vi "Benchmarking Asynchronous Calls.vi"() -> ()   [LabVIEW 2016]
doc: "This example requests web pages from the specified servers using an HTTP Get request and records how long the requests take. This example demonstrates and compares four different design patterns that accomplish this task:\n\n* Call By Reference node inside a For Loop to sequentially call the target VI\n* Call By Reference node inside a Parallel For Loop to allow some calls to execute in parallel depending on the number of CPU cores\n* Run VI method to execute all calls in parallel\n* Asynchronously calling VIs using the Start Asynchronous Call node to execute all calls in parallel\n\nIn general, if an application is I/O bound (ex: communication over the network), the parallel call approaches perform better. The default behavior of the Parallel For loop will run frames in parallel based on the number of CPU cores. The Run VI method and asynchronous call patterns allow a user to define the amount of parallelism at run time. \n\nIf an application is local CPU bound, the Parallel For Loop approach will perform the best. It utilizes the number of CPU cores and has less overhead when compared to the Run VI method and the asynchronous call pattern.\n\nThe actual performance results for this example depend largely on the computer and network connection.\n\nThe asynchronous call pattern and the Run VI method require overhead to allow the run-time defined parallelism. This overhead is negligible when compared to the I/O usage as in this example. The asynchronous call pattern has less overhead than the Run VI method. Depending on the application, the asynchronous call pattern might require LabVIEW to open fewer VI references and is more efficient when passing parameters to and from the target VI. The asynchronous call pattern also has a simpler syntax than the Run VI method."
panel:
  in  "Address":string="Address"
  out "Progress 3":i32(slide) scale=0.0..8.0
  out "Progress 2":i32(slide) scale=0.0..8.0
  out "Progress 1":i32(slide) scale=0.0..8.0
  out "Progress 0":i32(slide) scale=0.0..8.0
  out "Asynchronous Call By Reference":dbl
  out "Run VI Method":dbl
  out "Call By Reference (Parallel For Loop)":dbl
  out "Call By Reference":dbl
  # "Overview: Demonstrates the performance of Asynchronous VI Calls against other VI calling techniques.\nRequirements: A network connection\nInstructions:\nRun the VI. Observe the benchmark values below. Note that these times may be affected by network issues. See the block diagram for more information."
  # "Note: In general, if an application is I/O bound (communication over the network, e.g.), the parallel call approaches perform better. The default behavior of the Parallel For Loop will run frames in parallel based on the number of CPU cores. The Run VI method and asynchronous call patterns allow a user to define the amount of parallelism at run time. If an application is local CPU bound, the Parallel For Loop approach will perform the best. It utilizes the number of CPU cores and has less overhead when compared to the Run VI method and the asynchronous call pattern.\n\nThe asynchronous call pattern and the Run VI method require overhead to allow the run-time defined parallelism. This overhead is negligible when compared to the I/O usage as in this example. The asynchronous call pattern has less overhead than the Run VI method. Depending on the application, the asynchronous call pattern might require LabVIEW to open fewer VI references and is more efficient when passing parameters to and from the target VI. The asynchronous call pattern also has a simpler syntax than the Run VI method."
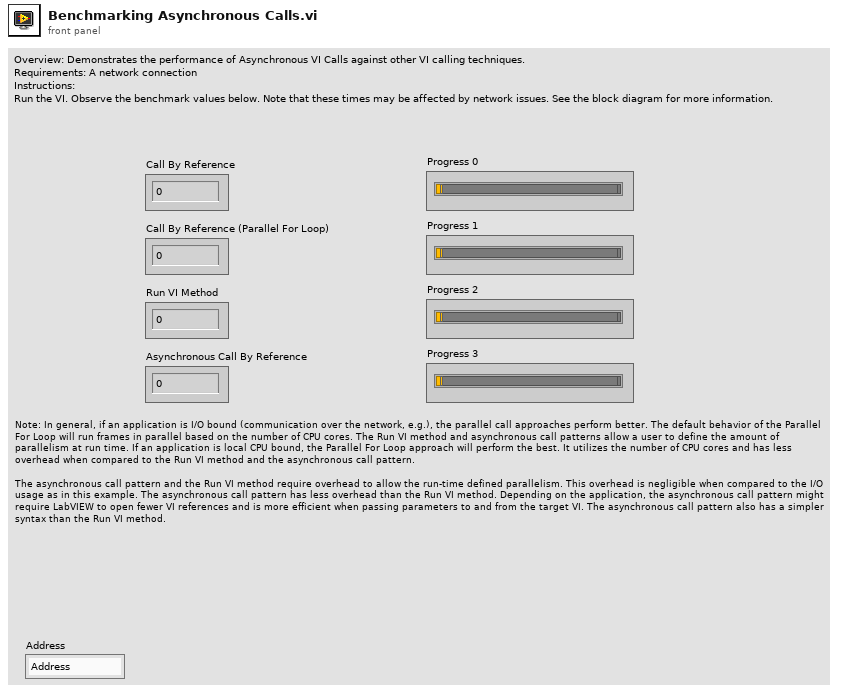
[diagram p1: front panel]
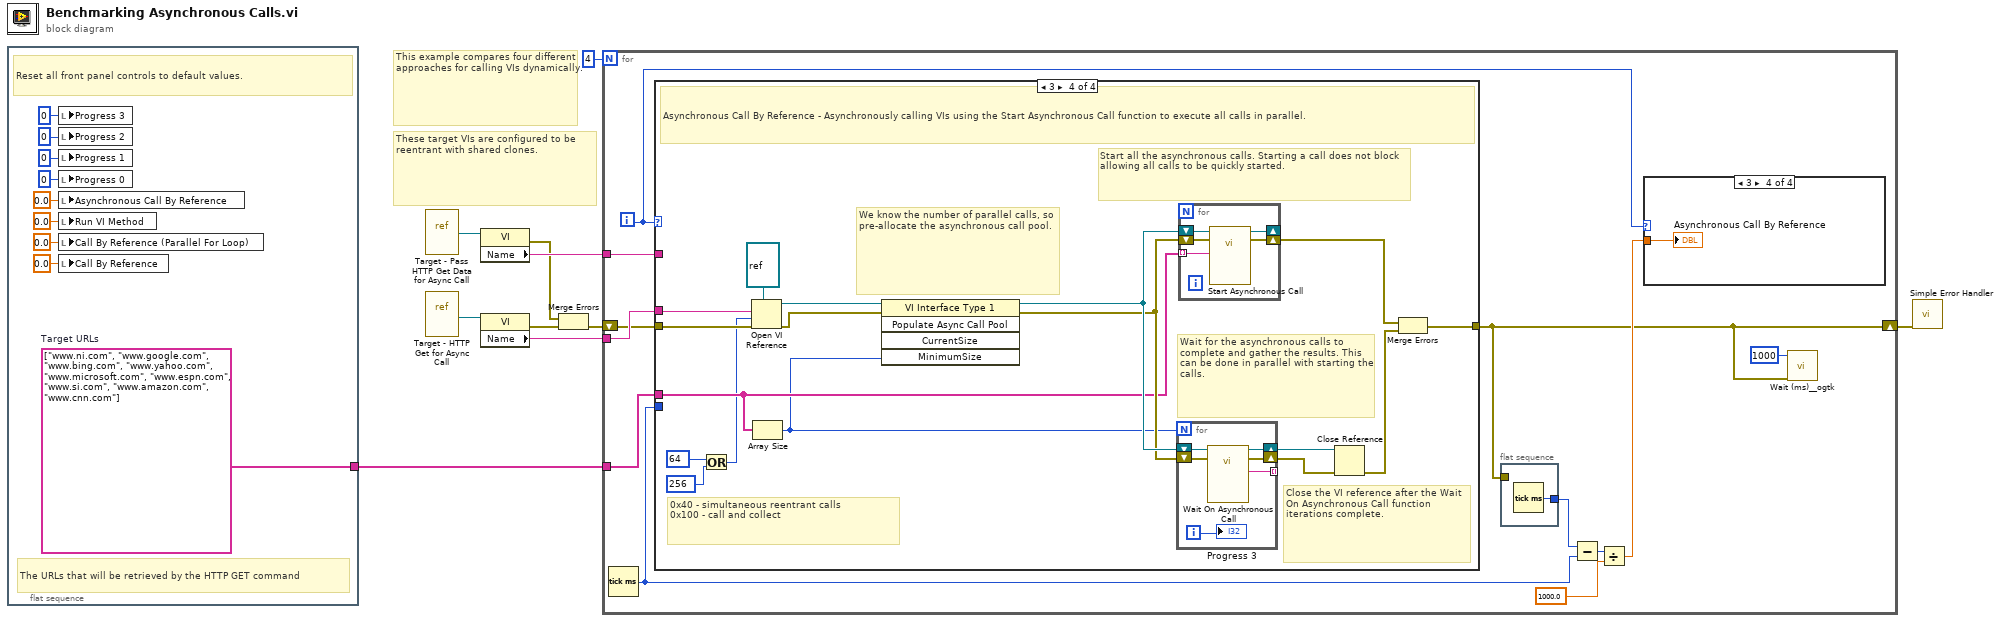
[diagram p0: block diagram]
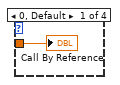
[diagram p2: hidden frame]
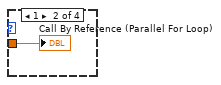
[diagram p3: hidden frame]
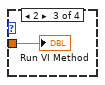
[diagram p4: hidden frame]
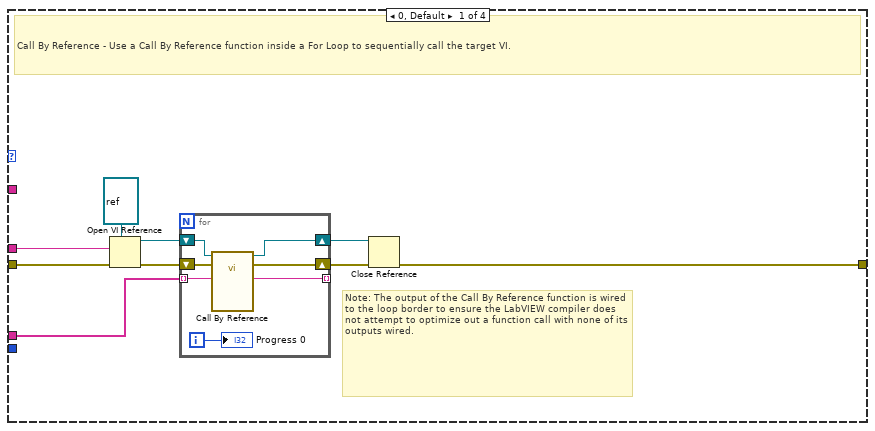
[diagram p5: hidden frame]
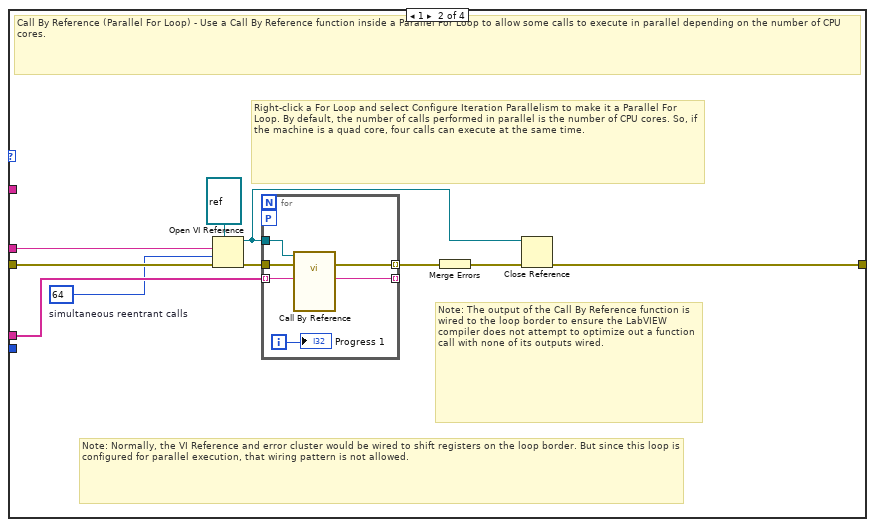
[diagram p6: hidden frame]
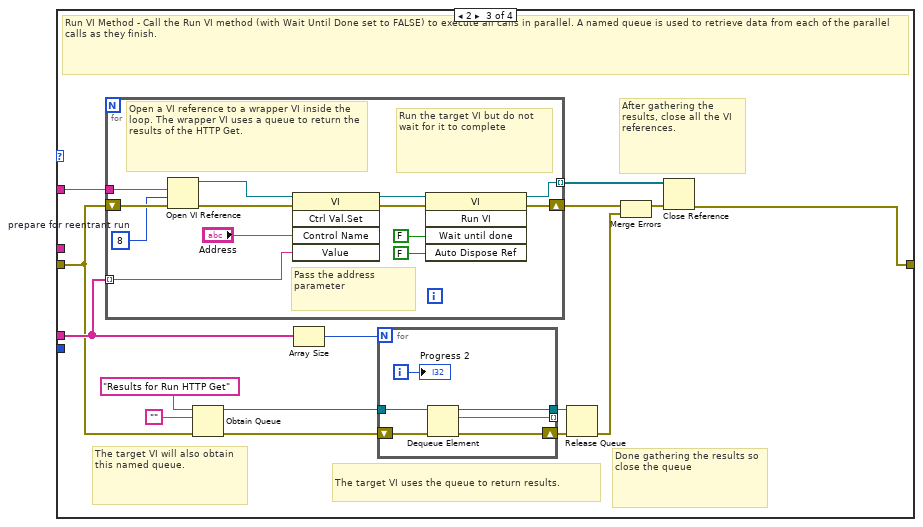
[diagram p7: hidden frame]
diagram:
  # "This example compares four different approaches for calling VIs dynamically."
  # "These target VIs are configured to be reentrant with shared clones."
  n1 = flat-sequence {
    tunnel: [w11] -> w1
    frame #0 {
      w11 = string[] ["www.ni.com", "www.google.com", "www.bing.com", "www.yahoo.com", "www.microsoft.com", "www.espn.com", "www.si.com", "www.amazon.com", "www.cnn.com"]  # Target URLs
      # "The URLs that will be retrieved by the HTTP GET command"
      # "Reset all front panel controls to default values."
      n2 = local write "Progress 3"(0 ("Progress 3")) -> ()
      n3 = local write "Progress 2"(0 ("Progress 2")) -> ()
      n4 = local write "Progress 1"(0 ("Progress 1")) -> ()
      n5 = local write "Progress 0"(0 ("Progress 0")) -> ()
      n6 = local write "Asynchronous Call By Reference"(0.0 ("Asynchronous Call By Reference")) -> ()
      n7 = local write "Run VI Method"(0.0 ("Run VI Method")) -> ()
      n8 = local write "Call By Reference (Parallel For Loop)"(0.0 ("Call By Reference (Parallel For Loop)")) -> ()
      n9 = local write "Call By Reference"(0.0 ("Call By Reference")) -> ()
    }
  }
  n10 = vi-ref "Target - Pass HTTP Get Data for Async Call.vi"() -> (w7:refnum<vi>)
  n11 = vi-ref "Target - HTTP Get for Async Call.vi"() -> (w10:refnum<vi>)
  n12 = property class="VI"(reference=w7) -> (error out=w2:errorcluster, "Name"=w6:string)  [unwired: 1 in, 1 out]
  n13 = property class="VI"(reference=w10) -> (error out=w8:errorcluster, "Name"=w9:string)  [unwired: 1 in, 1 out]
  n14 = Merge Errors(w2, w8) -> (w3:errorcluster)
  n15 = for {
    N: 4 -> [_]
    tunnel: w9 -> [w31]
    tunnel: w1 -> [w29]
    tunnel: w6 -> [w28]
    shift-right: [w21] -> w5
    shift-left: w3 -> [w30]
    i -> [w23]
    n16 = Tick Count (ms)() -> (millisecond timer value=w24:u32)
    n17 = case shown="3" w23 {
      tunnel: w31 -> [w45 w62 _ w119]
      tunnel: w30 -> [w44 w61 w69 w118]
      tunnel: w29 -> [w40 w59 w71 w111]
      tunnel: w24 -> [_ _ _ _]
      tunnel: [w37 w58 w72 w108] -> w21
      tunnel: w28 -> [_ _ w83 _]
      frame 0, Default {
        # "Note: The output of the Call By Reference function is wired to the loop border to ensure the LabVIEW compiler does not attempt to optimize out a function call with none of its outputs wired."
        # "Call By Reference - Use a Call By Reference function inside a For Loop to sequentially call the target VI."
        n18 = Open VI Reference(type specifier VI Refnum (for type only)=refnum<vi> refnum, vi path=w45, error in (no error)=w44) -> (vi reference=w42:refnum<vi>, error out=w41:errorcluster)  [unwired: 3 in]
        n19 = for {
          tunnel: w40 -> [w50] mode=indexing
          shift-right: [w49] -> w39
          shift-left: w42 -> [w52]
          shift-right: [w48] -> w38
          shift-left: w41 -> [w51]
          tunnel: [w47] -> _ mode=indexing
          i -> [w46]
          n20 = call-by-ref "?"(reference=w52, error in=w51, "Address"=w50) -> (reference out=w49:refnum<vi>, error out=w48:errorcluster, "Results"=w47:string)  [unwired: 10 in]
          "Progress 0" <- w46
        }
        n21 = Close Reference(reference=w39, error in (no error)=w38) -> (error out=w37:errorcluster)
      }
      frame 1 {
        w57 = 64  # simultaneous reentrant calls
        # "Note: Normally, the VI Reference and error cluster would be wired to shift registers on the loop border. But since this loop is configured for parallel execution, that wiring pattern is not allowed."
        # "Note: The output of the Call By Reference function is wired to the loop border to ensure the LabVIEW compiler does not attempt to optimize out a function call with none of its outputs wired."
        # "Right-click a For Loop and select Configure Iteration Parallelism to make it a Parallel For Loop. By default, the number of calls performed in parallel is the number of CPU cores. So, if the machine is a quad core, four calls can execute at the same time."
        # "Call By Reference (Parallel For Loop) - Use a Call By Reference function inside a Parallel For Loop to allow some calls to execute in parallel depending on the number of CPU cores."
        n22 = Open VI Reference(type specifier VI Refnum (for type only)=refnum<vi> refnum, vi path=w62, options=w57, error in (no error)=w61) -> (vi reference=w54:refnum<vi>, error out=w56:errorcluster)  [unwired: 2 in]
        n23 = for {
          tunnel: w59 -> [w68] mode=indexing
          tunnel: [w67] -> _ mode=indexing
          workers-P: _ -> [_]
          tunnel: w54 -> [w66]
          tunnel: w56 -> [w65]
          tunnel: [w64] -> w55 mode=indexing
          i -> [w63]
          n24 = call-by-ref "?"(reference=w66, error in=w65, "Address"=w68) -> (error out=w64:errorcluster, "Results"=w67:string)  [unwired: 10 in, 1 out]
          "Progress 1" <- w63
        }
        n25 = Merge Errors(w55) -> (w53:errorcluster)
        n26 = Close Reference(reference=w54, error in (no error)=w53) -> (error out=w58:errorcluster)
      }
      frame 2 {
        # "After gathering the results, close all the VI references."
        # "Done gathering the results so close the queue"
        # "The target VI uses the queue to return results."
        # "The target VI will also obtain this named queue."
        # "Run VI Method - Call the Run VI method (with Wait Until Done set to FALSE) to execute all calls in parallel. A named queue is used to retrieve data from each of the parallel calls as they finish."
        n27 = for {
          tunnel: w83 -> [w101]
          tunnel: w71 -> [w92] mode=indexing
          tunnel: [w91] -> w74 mode=indexing
          shift-right: [w90] -> w75
          shift-left: w69 -> [w102]
          w100 = 8  # prepare for reentrant run
          # "Open a VI reference to a wrapper VI inside the loop. The wrapper VI uses a queue to return the results of the HTTP Get."
          # "Pass the address parameter"
          # "Run the target VI but do not wait for it to complete"
          n28 = Open VI Reference(vi path=w101, options=w100, error in (no error)=w102) -> (vi reference=w97:refnum<vi>, error out=w96:errorcluster)  [unwired: 3 in]
          n29 = invoke class="VI" method="Ctrl Val.Set"(reference=w97, error in=w96, "Control Name"="Address", "Value"=w92) -> (reference out=w94:refnum<vi>, error out=w93:errorcluster)  [unwired: 1 in, 3 out]
          n30 = invoke class="VI" method="Run VI"(reference=w94, error in=w93, "Wait until done"=FALSE ("Wait Until Done"), "Auto Dispose Ref"=FALSE ("Auto Dispose Reference")) -> (reference out=w91:refnum<vi>, error out=w90:errorcluster)  [unwired: 1 in, 3 out]
        }
        n31 = Obtain Queue(name (unnamed)="Results for Run HTTP Get", element data type="", error in (no error)=w69) -> (queue out=w80:refnum<queue>, error out=w79:errorcluster)  [unwired: 2 in, 1 out]
        n32 = Array Size(array=w71) -> (size(s)=w70:i32)
        n33 = for {
          N: w70 -> [_]
          tunnel: w80 -> [w89]
          shift-right: [w85] -> w77
          shift-left: w79 -> [w88]
          tunnel: [w86] -> w78
          tunnel: [w87] -> _ mode=indexing
          i -> [w84]
          n34 = Dequeue Element(queue=w89, error in (no error)=w88) -> (queue out=w86:refnum<queue>, element=w87:string, error out=w85:errorcluster)  [unwired: 1 in, 1 out]
          "Progress 2" <- w84
        }
        n35 = Release Queue(queue=w78, error in (no error)=w77) -> (error out=w76:errorcluster)  [unwired: 1 in, 2 out]
        n36 = Merge Errors(w75, w76) -> (w73:errorcluster)
        n37 = Close Reference(reference=w74, error in (no error)=w73) -> (error out=w72:errorcluster)
      }
      frame 3 {
        # "Close the VI reference after the Wait On Asynchronous Call function iterations complete."
        # "Start all the asynchronous calls. Starting a call does not block allowing all calls to be quickly started."
        # "Wait for the asynchronous calls to complete and gather the results. This can be done in parallel with starting the calls."
        # "0x40 - simultaneous reentrant calls\n0x100 - call and collect"
        # "We know the number of parallel calls, so pre-allocate the asynchronous call pool."
        # "Asynchronous Call By Reference - Asynchronously calling VIs using the Start Asynchronous Call function to execute all calls in parallel."
        n38 = Or(x=64 ("options"), y=256 ("options")) -> (x .or. y?=w103:i32)
        n39 = Open VI Reference(type specifier VI Refnum (for type only)=refnum<vi> refnum, vi path=w119, options=w103, error in (no error)=w118) -> (vi reference=w115:refnum<vi>, error out=w114:errorcluster)  [unwired: 2 in]
        n40 = Array Size(array=w111) -> (size(s)=w106:i32)
        n41 = invoke class="VI Interface Type 1" method="Populate Async Call Pool"(reference=w115, error in=w114, "MinimumSize"=w106) -> (reference out=w113:refnum<vi>, error out=w112:errorcluster)  [unwired: 2 in, 3 out]
        n42 = for {
          N: w106 -> [_]
          shift-right: [w123] -> w116
          shift-left: w113 -> [w125]
          shift-right: [w122] -> w107
          shift-left: w112 -> [w124]
          tunnel: [w120] -> _ mode=indexing
          i -> [w121]
          n43 = call-by-ref "Wait On Asynchronous Call"(reference=w125, error in=w124) -> (reference out=w123:refnum<vi>, error out=w122:errorcluster, "Results"=w120:string)  [unwired: 11 in]
          "Progress 3" <- w121
        }
        n44 = for {
          tunnel: w111 -> [w128] mode=indexing
          shift-right: [w129] -> w110
          shift-left: w112 -> [w130]
          shift-right: [w126] -> _
          shift-left: w113 -> [w127]
          n45 = call-by-ref "Start Asynchronous Call"(reference=w127, error in=w130, "Address"=w128) -> (reference out=w126:refnum<vi>, error out=w129:errorcluster)  [unwired: 10 in, 1 out]
        }
        n46 = Close Reference(reference=w116, error in (no error)=w107) -> (error out=w109:errorcluster)
        n47 = Merge Errors(w110, w109) -> (w108:errorcluster)
      }
    }
    n48 = flat-sequence {
      tunnel: w21 -> [_]
      tunnel: [w36] -> w25
      frame #0 {
        n49 = Tick Count (ms)() -> (millisecond timer value=w36:u32)
      }
    }
    n50 = Subtract(x=w25, y=w24) -> (x-y=w27:u32)
    n51 = Divide(x=w27, y=1000.0) -> (x/y=w22:dbl)
    n52 = case shown="3" w23 {
      tunnel: w22 -> [w32 w33 w34 w35]
      frame 0, Default {
        "Call By Reference" <- w32
      }
      frame 1 {
        "Call By Reference (Parallel For Loop)" <- w33
      }
      frame 2 {
        "Run VI Method" <- w34
      }
      frame 3 {
        "Asynchronous Call By Reference" <- w35
      }
    }
    n53 = call <userlib>:"Wait (ms)__ogtk.vi"("error in (no error)"=w21, "milliseconds to wait"=u32 1000) -> ()  [unwired: 8 in, 2 out]
  }
  n54 = call <vilib>:"Simple Error Handler.vi"("error in (no error)"=w5) -> ()  [unwired: 4 in, 5 out]
